vi "SaveDataAcqCont.vi"(8 "Boolean in":refnum<vi>, 9 "Array in":T1[](array[typedef]), 10 "Location":T3, 11 "Type of scan":T2) -> (1 "Array out":T1[](array[typedef]), 3 "Aborted":bool)   [LabVIEW 2022 SP3]
uses:
  Controls/location.ctl
  Controls/ScanType2.ctl
  Controls/ScanParams.ctl
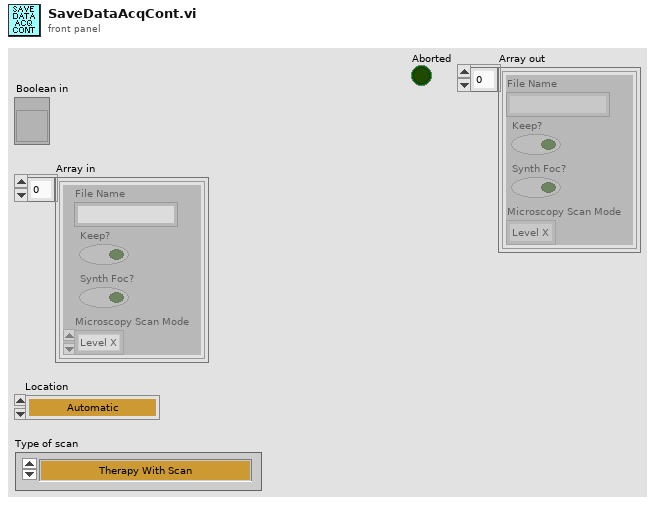
[diagram p1: front panel]
types:
  T1 = typedef "ScanParams.ctl" = cluster{"File Name":string, "Keep?":bool, "Synth Foc?":bool, "Microscopy Scan Mode":enum32{"Level X", "Level Y", "Overview Scan", "Detailed Scan", "V-Z Scan"}}
  T2 = typedef "ScanType2.ctl" = enum16{"Therapy With Scan", "M scan", "M Scan With Therapy Burst", "1-D B Scan", "1-D B Scan With Therapy Burst", "2-D B Scan", "2-D B Scan With Therapy Burst", "Rotational Scan", "1-D B-Scan PRF", "2-D B-Scan PRF", "Real-Time Scan", "Contrast Agents", "1-D w/ Real-Time Set Up", "Dual Transducer", "Acoustic Microscopy", "Hydrophone Scanning"}
  T3 = typedef "location.ctl" = enum16{"Automatic", "WCM Main", "Hawaii", "Columbia MM3000", "Columbia  NI System", "NYU", "RRI 2", "UHI Allen", "CUMC RT", "Chiba", "Stony Brook", "WCM Microscopy", "WCM Aeoretch", "WCM Optics Lab", "WCM Main 2Axis", "WCM Rotation", "WCM SAM SMAC", "SERI GP"}
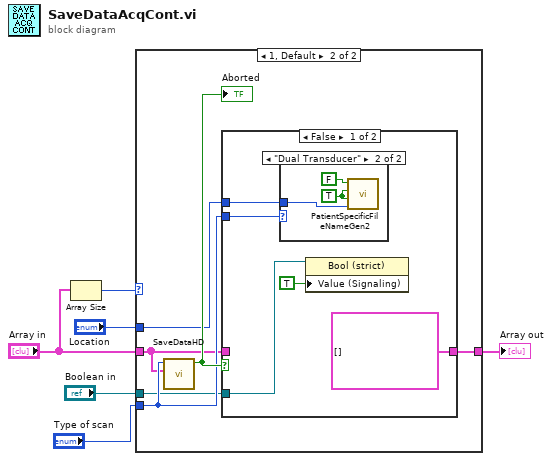
[diagram p0: block diagram]
diagram:
  n1 = Array Size(array="Array in") -> (size(s)=w4:i32)
  n2 = case shown="1, Default" w4 {
    tunnel: "Type of scan" -> [_ w11]
    tunnel: "Array in" -> [w7 w8]
    tunnel: "Location" -> [_ w12]
    tunnel: "Boolean in" -> [_ w10]
    tunnel: [w7 w9] -> w1
    frame 0 {
    }
    frame 1, Default {
      n3 = call "SaveDataHD.vi"("Array"=w8, "Type of scan"=w11) -> ("Aborted"=w13:bool)  [unwired: 5 in, 4 out]
      "Aborted" <- w13
      n4 = case shown="False" w13 {
        tunnel: w12 -> [w17 _]
        tunnel: w11 -> [w16 _]
        tunnel: w10 -> [w15 _]
        tunnel: [T1[] [] w22] -> w9
        tunnel: w8 -> [_ w22]
        frame False {
          n5 = case shown="\"Dual Transducer\"" w16 {
            tunnel: w17 -> [_ w19]
            frame "M scan", Default {
            }
            frame "Dual Transducer" {
              w20 = TRUE ("Add to Database")
              n6 = call "PatientSpecificFileNameGen2.vi"("Location"=w19, "Add to Database"=w20, "Done"=w20, "Auto Increment"=FALSE) -> ()  [unwired: 2 out]
            }
          }
          n7 = property on="Property Node" class="Bool (strict)"(reference=w15, "Value (Signaling)"=TRUE) -> ()  [unwired: 1 in, 2 out]
        }
        frame True {
        }
      }
    }
  }
  "Array out" <- w1
